vi "Initialize--Method.vi"(8 "error in (no error)":errorcluster, 10 "VISA Resource":refnum<visa-resource-name>, 11 "Watlow F4T in":refnum<class "Watlow F4T.lvclass">) -> (0 "error out":errorcluster, 2 "Connected?":bool, 3 "Watlow F4T out":refnum<class "Watlow F4T.lvclass">)   [LabVIEW 2024, in "Watlow F4T.lvclass"]
uses:
  Watlow F4T.lvclass
  Process Controller/Controls/Temperature Units--Enum.ctl
  Process Controller/Controls/Limits--Cluster.ctl
  Process Controller/Controls/Temp Ramp Rate Data--Cluster.ctl
  Process Controller/Controls/Rate Units--Enum.ctl
  Process Controller/Controls/Temp Data--Cluster.ctl
  Watlow F4T.lvclass/Watlow F4T.ctl
  Process Controller/_Thermal Process Controller.lvclass
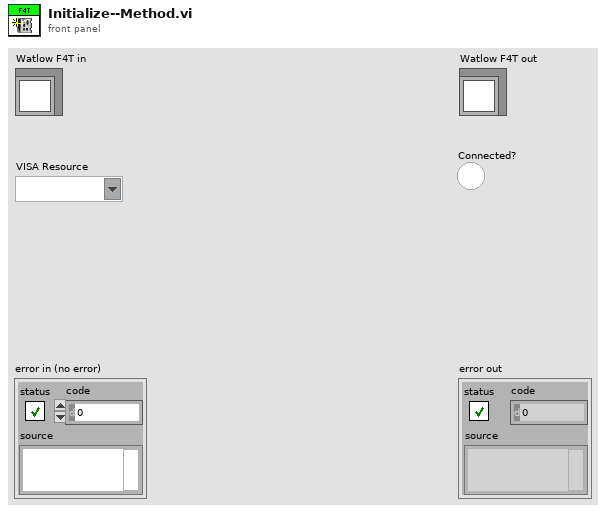
[diagram p1: front panel]
types:
  T1 = typedef "_Thermal Process Controller.lvclass/Temp Data--Cluster.ctl" = cluster{"Temp":dbl, "Temp Units":T2}
  T2 = typedef "_Thermal Process Controller.lvclass/Temperature Units--Enum.ctl" = enum16{"Degrees F", "Degrees C", "Degrees K"}
  T3 = typedef "_Thermal Process Controller.lvclass/Temp Ramp Rate Data--Cluster.ctl" = cluster{"Temp Ramp Rate":dbl, "Temp Units":T2, "Rate Units":T4}
  T4 = typedef "_Thermal Process Controller.lvclass/Rate Units--Enum.ctl" = enum16{"Degrees/Minutes", "Degrees/Hours"}
  T5 = typedef "_Thermal Process Controller.lvclass/Limits--Cluster.ctl" = cluster{"Upper Limit":dbl, "Lower Limit":dbl}
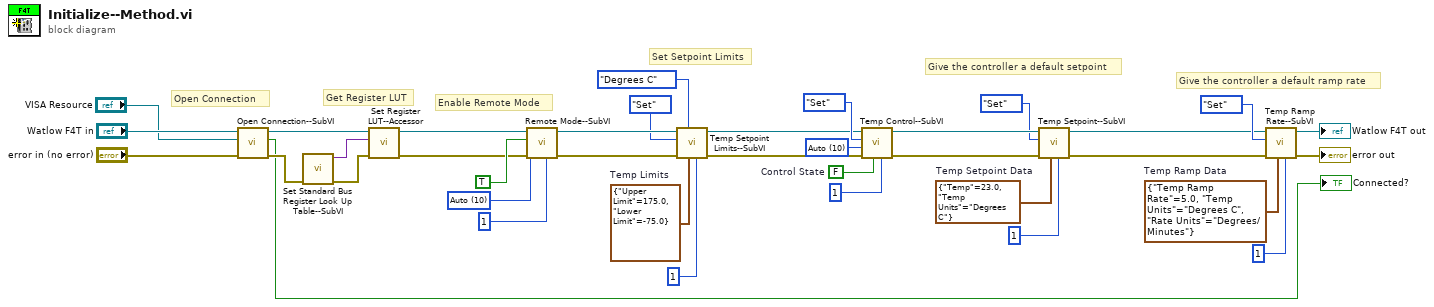
[diagram p0: block diagram]
diagram:
  w37 = u16 10 items=["Off"=62, "Auto"=10, "Manual"=54] ("Control Mode (Auto)")
  w34 = u16 10 items=["Auto"=10, "Manual"=54] ("Mode")
  w16 = FALSE  # Control State
  w20 = T1 {"Temp"=23.0, "Temp Units"=enum."Degrees C"}  # Temp Setpoint Data
  w26 = T3 {"Temp Ramp Rate"=5.0, "Temp Units"=enum."Degrees C", "Rate Units"=enum."Degrees/Minutes"}  # Temp Ramp Data
  w7 = T5 {"Upper Limit"=175.0, "Lower Limit"=-75.0}  # Temp Limits
  # "Enable Remote Mode"
  # "Open Connection"
  # "Give the controller a default ramp rate"
  # "Give the controller a default setpoint"
  # "Set Setpoint Limits"
  # "Get Register LUT"
  n1 = call "Open Connection--SubVI.vi"("error in (no error)"="error in (no error)", "VISA Refnum in"="VISA Resource", "Watlow F4T in"="Watlow F4T in") -> ("error out"=w13:errorcluster, "IsConnected"=→"Connected?":bool, "Watlow F4T out"=w32:refnum<class "Watlow F4T.lvclass">)  [unwired: 6 in]
  n2 = call "Set Standard Bus Register Look Up Table--SubVI.vi"("error in"=w13) -> ("error out"=w12:errorcluster, "Standard Bus Register Look Up Table"=w11:variant)  [unwired: 9 in]
  n3 = call "Set Register LUT--Accessor.vi"("error in (no error)"=w12, "Register LUT"=w11, "Watlow F4T in"=w32) -> ("error out"=w27:errorcluster, "Watlow F4T out"=w28:refnum<class "Watlow F4T.lvclass">)  [unwired: 7 in]
  n4 = call "Remote Mode--SubVI.vi"("Instance"=1, "error in"=w27, "Mode (Auto)"=w34, "Enable (T)"=TRUE, "Watlow F4T in"=w28) -> ("error out"=w30:errorcluster, "Watlow F4T out"=w29:refnum<class "Watlow F4T.lvclass">)  [unwired: 5 in]
  n5 = call "Temp Setpoint Limits--SubVI.vi"("Instance(1)"=1, "Limits"=w7, "Temp Units"=Temperature_Units--Enum."Degrees C", "error in (no error)"=w30, "Get/Set"=enum16{"Get", "Set"}."Set", "Watlow F4T in"=w29) -> ("error out"=w14:errorcluster, "Watlow F4T out"=w15:refnum<class "Watlow F4T.lvclass">)  [unwired: 4 in]
  n6 = call "Temp Control--SubVI.vi"("Instance"=1, "Temp Control in"=w16, "error in"=w14, "Control Mode (Auto)"=w37, "Get/Set"=enum16{"Get", "Set"}."Set", "Watlow F4T in"=w15) -> ("error out"=w35:errorcluster, "Watlow F4T out"=w36:refnum<class "Watlow F4T.lvclass">)  [unwired: 3 in, 1 out]
  n7 = call "Temp Setpoint--SubVI.vi"("Instance(1)"=1, "Temp Setpoint Data"=w20, "error in (no error)"=w35, "Get/Set"=enum16{"Get", "Set"}."Set", "Watlow F4T In"=w36) -> ("error out"=w22:errorcluster, "Watlow F4T out"=w21:refnum<class "Watlow F4T.lvclass">)  [unwired: 4 in, 1 out]
  n8 = call "Temp Ramp Rate--SubVI.vi"("Instance(1)"=1, "Temp Ramp Data"=w26, "error in (no error)"=w22, "Get/Set"=enum16{"Get", "Set"}."Set", "Watlow F4T in"=w21) -> ("error out"=→"error out":errorcluster, "Watlow F4T out"=→"Watlow F4T out":refnum<class "Watlow F4T.lvclass">)  [unwired: 4 in, 1 out]
